vi "Update Layout.vi"(7 "Page Size":dbl, 8 "error in (no error)":errorcluster, 10 "UI Refs":T1, 11 "ArrayManager in":refnum<class "ArrayManager.lvclass">) -> (0 "error out":errorcluster, 3 "ArrayManager out":refnum<class "ArrayManager.lvclass">)   [LabVIEW 2020, in "OOPanel.lvlib" / "ArrayManager.lvclass"]
uses:
  ArrayManager.lvclass
  UI Refs.ctl
  ArrayManager.lvclass/ArrayManager.ctl
  ArrayPanel/ArrayPanel.lvclass
  C:/dev/LabVIEW/lv-oopanel/OOPanel/Panel/Panel.lvclass
  Manager/Manager.lvclass
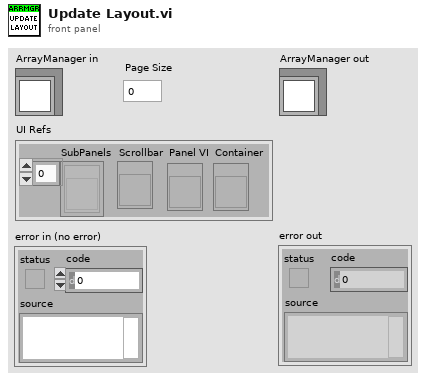
[diagram p1: front panel]
types:
  T1 = typedef "OOPanel.lvlib/ArrayManager.lvclass/UI Refs.ctl" = cluster{"SubPanels":refnum<vi>[], "Scrollbar":refnum<vi>, "Panel VI":refnum<vi>, "Container":refnum<vi>}
  T2 = typedef "OOPanel.lvlib/ArrayPanel.lvclass/Desired Size.ctl" = cluster{"Width":u32, "Height":u32}
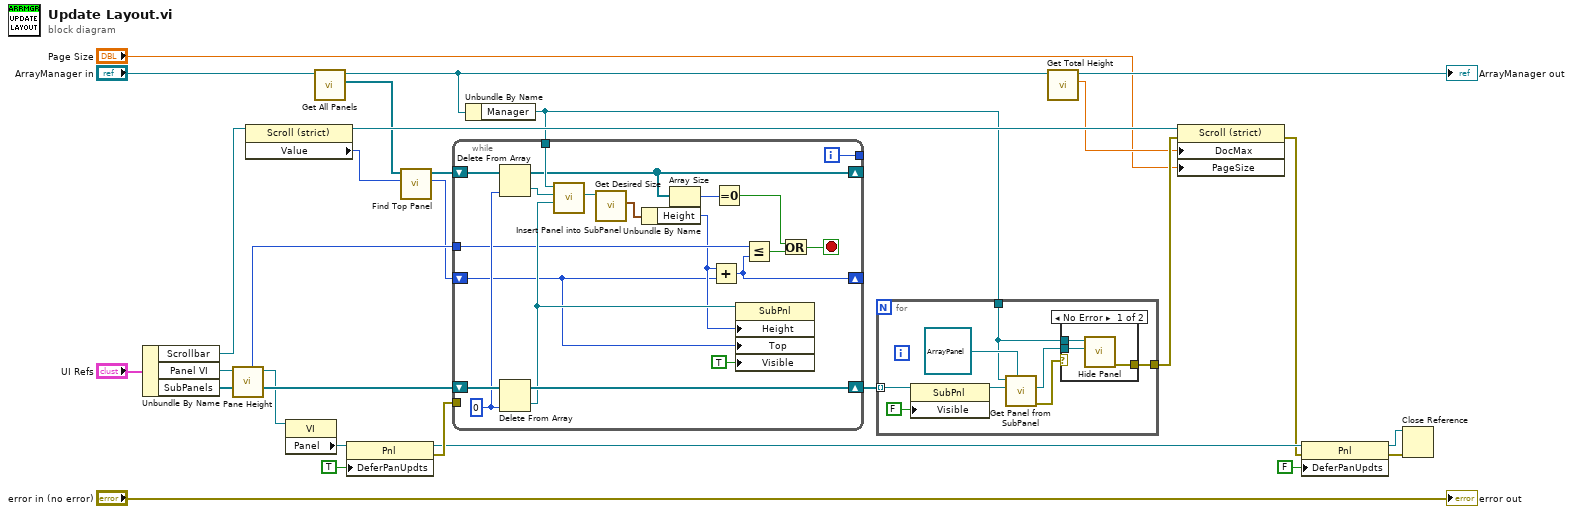
[diagram p0: block diagram]
diagram:
  n1 = Unbundle By Name("UI Refs") -> ("Scrollbar"=w25:refnum<vi>, "Panel VI"=w21:refnum<vi>, "SubPanels"=w23:refnum<vi>[])
  n2 = call "Pane Height.vi"("Panel VI in"=w21) -> ("Panel VI"=w20:refnum<vi>, "Height"=w22:u32)  [unwired: 9 in]
  n3 = property class="Scroll (strict)"(reference=w25) -> (reference out=w24:refnum<vi>, "Value"=w2:i32)  [unwired: 1 in, 1 out]
  n4 = property class="VI"(reference=w20) -> ("Panel"=w19:refnum<vi>)  [unwired: 1 in, 2 out]
  n5 = call "Get All Panels.vi"("PanelArray in"="ArrayManager in") -> ("Panels"=w4:refnum<class "ArrayPanel.lvclass">[], "PanelArray out"=w8:refnum<class "ArrayManager.lvclass">)  [unwired: 8 in, 1 out]
  n6 = property class="Pnl"(reference=w19, "DeferPanUpdts"=TRUE ("Defer Panel Updates")) -> (reference out=w15:refnum<vi>, error out=w17:errorcluster)  [unwired: 1 in]
  n7 = call "Find Top Panel.vi"("Scroll"=w2, "All Panels"=w4) -> ("Start"=w1:i32, "Panels"=w3:refnum<class "ArrayPanel.lvclass">[])  [unwired: 8 in]
  n8 = Unbundle By Name(w8) -> ("Manager"=w9:refnum<class "Manager.lvclass">)
  n9 = while {
    shift-right: [w47] -> w10
    shift-left: w23 -> [w48]
    tunnel: w22 -> [w38]
    tunnel: w17 -> [_]
    shift-right: [w34] -> _
    shift-left: w3 -> [w46]
    tunnel: w9 -> [w44]
    shift-right: [w37] -> _
    shift-left: w1 -> [w29]
    tunnel: [w35] -> _
    i -> [w35]
    stop <- w32 stop-if-true
    w45 = 0 ("index")
    n10 = Delete From Array(array=w46, index=w45) -> (deleted portion=w43:refnum<class "ArrayPanel.lvclass">, array with subset deleted=w34:refnum<class "ArrayPanel.lvclass">[])  [unwired: 1 in]
    n11 = Delete From Array(array=w48, index=w45) -> (deleted portion=w42:refnum<vi>, array with subset deleted=w47:refnum<vi>[])  [unwired: 1 in]
    n12 = call "Insert Panel into SubPanel.vi"("SubPanel"=w42, "Panel In"=w43, "Manager in"=w44) -> ("Panel"=w40:refnum<class "ArrayPanel.lvclass">)  [unwired: 6 in, 2 out]
    n13 = call-dynamic "Get Desired Size.vi"("ArrayPanel in"=w40) -> ("Desired Size"=w39:T2)  [unwired: 8 in, 2 out]
    n14 = Unbundle By Name(w39) -> ("Height"=w30:u32)
    n15 = Array Size(array=w34) -> (size(s)=w33:i32)
    n16 = Add(x=w30, y=w29) -> (x+y=w37:u32)
    n17 = Equal To 0?(x=w33) -> (x = 0?=w31:bool)
    n18 = property class="SubPnl"(reference=w42, "Height"=w30, "Top"=w29, "Visible"=TRUE) -> ()  [unwired: 1 in, 2 out]
    n19 = Less Or Equal?(x=w38, y=w37) -> (x <= y?=w36:bool)
    n20 = Or(x=w31, y=w36) -> (x .or. y?=w32:bool)
  }
  n21 = for {
    tunnel: w10 -> [w52] mode=indexing
    tunnel: w9 -> [w53]
    tunnel: [w49] -> w28
    n22 = property class="SubPnl"(reference=w52, "Visible"=FALSE) -> (reference out=w51:refnum<vi>)  [unwired: 1 in, 1 out]
    n23 = call "Get Panel from SubPanel.vi"("Panel Type (Panel)"=refnum<class "ArrayPanel.lvclass"> refnum ("OOPanel.lvlib:ArrayPanel.lvclass"), "SubPanel"=w51, "Manager in"=w53) -> ("error out"=w55:errorcluster, "Panel"=w54:refnum<class "ArrayPanel.lvclass">)  [unwired: 6 in, 1 out]
    n24 = case shown="No Error" w55 {
      tunnel: w54 -> [w59 _]
      tunnel: w53 -> [w58 _]
      tunnel: [w57 _] -> w49
      frame No Error {
        n25 = call "Hide Panel.vi"("Panel In"=w59, "Manager in"=w58) -> ("error out"=w57:errorcluster)  [unwired: 7 in, 2 out]
      }
      frame Error {
      }
    }
  }
  n26 = call "Get Total Height.vi"("ArrayManager in"=w8) -> ("Total Height"=w6:dbl, "ArrayManager out"=→"ArrayManager out":refnum<class "ArrayManager.lvclass">)  [unwired: 8 in, 1 out]
  n27 = property class="Scroll (strict)"(reference=w24, error in=w28, "DocMax"=w6, "PageSize"="Page Size") -> (error out=w13:errorcluster)  [unwired: 1 out]
  n28 = property class="Pnl"(reference=w15, error in=w13, "DeferPanUpdts"=FALSE ("Defer Panel Updates")) -> (reference out=w11:refnum<vi>, error out=w12:errorcluster)
  n29 = Close Reference(reference=w11, error in (no error)=w12) -> ()  [unwired: 1 out]
  "error out" <- "error in (no error)"
